vi "ciclo4.vi"() -> ()   [LabVIEW 2011]
panel:
  out "Repeticiones":dbl
  out "Menor":dbl
  out "Mayor":dbl
  out "Promedio":dbl
  out "Temperatura":i32(slide) scale=0.0..60.0
  # "Generar 10 temperaturas, y al final presentar la temperatura mayor, menor y la temperatura promedio"
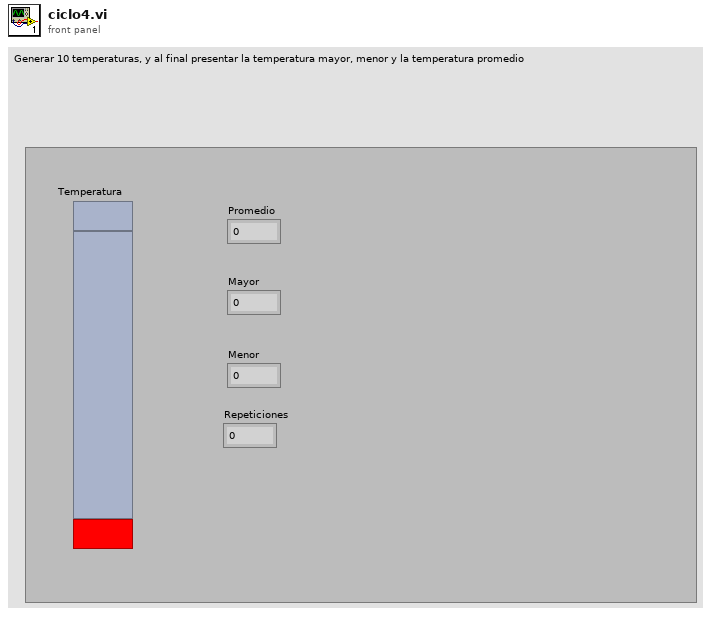
[diagram p1: front panel]
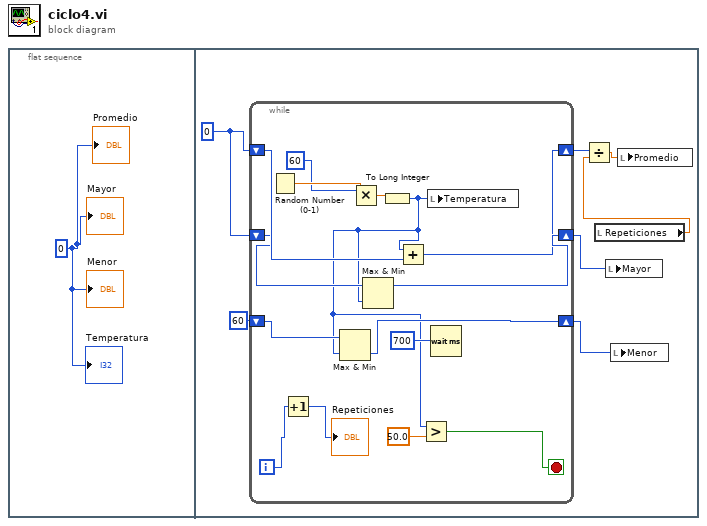
[diagram p0: block diagram]
diagram:
  n1 = flat-sequence {
    frame #0 {
      w1 = 0
      "Temperatura" <- w1
      "Promedio" <- w1
      "Mayor" <- w1
      "Menor" <- w1
    }
    frame #1 {
      w5 = 0
      n2 = while {
        shift-right: [w17] -> w8
        shift-left: w5 -> [w20]
        shift-right: [w18] -> w6
        shift-left: w5 -> [w14]
        shift-right: [w16] -> w4
        shift-left: 60 -> [w15]
        i -> [w10]
        stop <- w13 stop-if-true
        n3 = Random Number (0-1)() -> (number: 0 to 1=w23:dbl)
        n4 = Increment(x=w10) -> (x+1=→"Repeticiones":i32)
        n5 = Multiply(x=60, y=w23) -> (x*y=w21:dbl)
        n6 = To Long Integer(number=w21) -> (32bit integer=w11:i32)
        n7 = Max & Min(x=w15, y=w11) -> (min(x,y)=w16:i32)  [unwired: 1 out]
        n8 = Max & Min(x=w14, y=w11) -> (max(x,y)=w18:i32)  [unwired: 1 out]
        n9 = Add(x=w11, y=w20) -> (x+y=w17:i32)
        n10 = Greater?(x=w11, y=50.0) -> (0:w13:bool)
        n11 = local write "Temperatura"(w11) -> ()
        n12 = Wait (ms)(milliseconds to wait=u32 700 ("millisecond timer value")) -> ()  [unwired: 1 out]
      }
      n13 = local read "Repeticiones"() -> (w2:dbl)
      n14 = Divide(x=w8, y=w2) -> (x/y=w7:dbl)
      n15 = local write "Mayor"(w6) -> ()
      n16 = local write "Menor"(w4) -> ()
      n17 = local write "Promedio"(w7) -> ()
    }
  }
